vi "输入数据解析.vi"(0 "单个参数补充":dbl, 1 "从板号":dbl=1.0, 2 "主板二维码":string="BNET01", 3 "从板二维码":string="BNET01", 5 "主板引用":refnum<vi>, 7 "从板引用":refnum<vi>, 9 "主板选项":string="三级故障阀值", 11 "枚举":enum16{"主板", "从板"}(ring), 12 "快换":bool caption="快换写入") -> (4 "输出数组":dbl[][](array[numeric]), 6 "数组长度":dbl[](array[numeric]), 8 "循环次数":i32, 10 "命令":u32, 14 "名称":string[](array[string]), 15 "命令序号":u32[](array[numeric]))   [LabVIEW 2013] (continued)
                    n7568 = Quotient & Remainder(x=w19474, y=w19492) -> (x-y*floor(x/y)=w19491:dbl, floor(x/y)=w19495:dbl)
                    n7569 = Quotient & Remainder(x=w19473, y=w19487) -> (x-y*floor(x/y)=w19483:dbl, floor(x/y)=w19484:dbl)
                    n7570 = Quotient & Remainder(x=w19495, y=w19492) -> (x-y*floor(x/y)=w19490:dbl, floor(x/y)=w19494:dbl)
                    n7571 = Quotient & Remainder(x=w19484, y=w19487) -> (x-y*floor(x/y)=w19482:dbl, floor(x/y)=w19485:dbl)
                    n7572 = Quotient & Remainder(x=w19494, y=w19492) -> (x-y*floor(x/y)=w19489:dbl, floor(x/y)=w19493:dbl)
                    n7573 = Quotient & Remainder(x=w19485, y=w19487) -> (x-y*floor(x/y)=w19481:dbl, floor(x/y)=w19486:dbl)
                    n7574 = Quotient & Remainder(x=w19493, y=w19492) -> (x-y*floor(x/y)=w19488:dbl)  [unwired: 1 out]
                    n7575 = Quotient & Remainder(x=w19486, y=w19487) -> (x-y*floor(x/y)=w19480:dbl)  [unwired: 1 out]
                    n7576 = Build Array(w19488, w19489, w19490, w19491, w19480, w19481, w19482, w19483) -> (w19496:dbl[])
                  }
                  frame 3 {
                    w19504 = 256.0 ("y")
                    # "充电次数"
                    n7577 = Unbundle By Name(w19509) -> ("充电次数"=w19508:dbl, "应用车型"=w19506:dbl, "电池包组号"=w19505:dbl)
                    n7578 = Quotient & Remainder(x=w19508, y=w19504) -> (x-y*floor(x/y)=w19510:dbl, floor(x/y)=w19507:dbl)
                    n7579 = Quotient & Remainder(x=w19506, y=w19504) -> (x-y*floor(x/y)=w19502:dbl, floor(x/y)=w19503:dbl)
                    n7580 = Quotient & Remainder(x=w19505, y=w19504) -> (x-y*floor(x/y)=w19500:dbl, floor(x/y)=w19501:dbl)
                    n7581 = Build Array(w19507, w19510, w19503, w19502, w19501, w19500) -> (w19511:dbl[])
                  }
                  frame 4 {
                    # "SOC"
                    n7582 = Unbundle By Name(w19520) -> ("SOC"=w19519:dbl)
                    n7583 = call "输入分辨率计算-EV05.vi"("1字节?"=FALSE, "数值"=w19519, "分辨率"=0.1) -> ("低字节"=w19515:dbl, "高字节1"=w19516:dbl)  [unwired: 2 in, 5 out]
                    n7584 = Build Array(w19516, w19515) -> (w19521:dbl[])
                  }
                  frame 5 {
                    # "车牌号"
                    n7585 = Unbundle By Name(w19528) -> ("车牌号"=w19527:string)
                    n7586 = String To Byte Array(string=w19527) -> (unsigned byte array=w19531:u8[])
                    n7587 = Array Subset(array=w19531, length=8 ("长度")) -> (w19526:u8[])  [unwired: 1 in]
                  }
                  frame 6 {
                    n7588 = Unbundle By Name(w19549) -> ("最大允许单体电压"=w19547:dbl, "最大允许总电压"=w19546:dbl, "最大允许温度"=w19545:dbl, "最小允许温度"=w19544:dbl, "最大允许充电电流"=w19543:dbl, "最小允许充电电流"=w19542:dbl, "电流步长"=w19538:dbl, "最小允许单体电压"=w19541:dbl)
                    n7589 = call "输入分辨率计算-EV05.vi"("1字节?"=FALSE, "数值 2"=w19541, "数值"=w19547, "分辨率"=0.001) -> ("低字节 2"=w19533:dbl, "高字节 2"=w19534:dbl, "低字节"=w19557:dbl, "高字节1"=w19558:dbl)  [unwired: 1 in, 3 out]
                    n7590 = call "输入分辨率计算-EV05.vi"("1字节?"=FALSE, "数值"=w19546, "分辨率"=0.1) -> ("低字节"=w19555:dbl, "高字节1"=w19556:dbl)  [unwired: 2 in, 5 out]
                    n7591 = call "输入分辨率计算-EV05.vi"("1字节?"=TRUE, "数值 2"=w19544, "数值"=w19545, "偏移量"=-40.0, "分辨率"=1.0) -> ("高字节 2"=w19550:dbl, "高字节1"=w19554:dbl)  [unwired: 5 out]
                    n7592 = call "输入分辨率计算-EV05.vi"("1字节?"=FALSE, "数值 2"=w19542, "数值"=w19543, "偏移量"=0.0, "分辨率"=0.1) -> ("低字节 2"=w19539:dbl, "高字节 2"=w19540:dbl, "低字节"=w19552:dbl, "高字节1"=w19553:dbl)  [unwired: 3 out]
                    n7593 = Quotient & Remainder(x=w19538, y=256.0) -> (x-y*floor(x/y)=w19535:dbl, floor(x/y)=w19536:dbl)
                    n7594 = Build Array(w19558, w19557, w19556, w19555, w19554, w19550, w19553, w19552, w19540, w19539, w19536, w19535, w19534, w19533) -> (w19551:dbl[])
                  }
                }
              }
            }
          }
        }
        frame "电池包序号" {
          n7595 = case shown="真" w19573 {
            tunnel: [_ w19584] -> w19577
            tunnel: [_ w19583] -> w19576
            tunnel: w19575 -> [_ w19579]
            tunnel: [_ w19582] -> w19574
            tunnel: [_ u32 35 ("命令序号")] -> w19572
            frame False {
            }
            frame True {
              n7596 = Unbundle By Name(w19579) -> ("电池组信息(从板)"=w19580:refnum<vi>)
              n7597 = property class="Clust (严格)"(reference=w19580) -> ("Value"=w19578:T9)  [unwired: 1 in, 2 out]
              n7598 = for {
                N: 1 -> [_]
                tunnel: [w19590] -> w19584 mode=indexing
                tunnel: [w19589] -> w19583 mode=indexing
                tunnel: w19578 -> [w19588]
                tunnel: [w19587] -> w19582 mode=indexing
                i -> [w19586]
                n7599 = case shown="0, 默认" w19586 {
                  tunnel: [4 ("单个参数补充") 30 ("单个参数补充") 8 ("单个参数补充") 6 ("单个参数补充") 4 ("单个参数补充") 8 ("单个参数补充") 14 ("单个参数补充")] -> w19590
                  tunnel: [u32 2 ("命令序号") u32 1 ("命令序号") u32 3 ("命令序号") u32 4 ("命令序号") u32 5 ("命令序号") u32 6 ("命令序号") u32 7 ("命令序号")] -> w19589
                  tunnel: w19588 -> [w19598 w19614 w19626 w19655 w19665 w19672 w19692]
                  tunnel: [w19591 w19616 w19643 w19657 w19666 w19670 w19694] -> w19587
                  frame 0, Default {
                    n7600 = Unbundle By Name(w19598) -> ("电池包序号"=w19595:dbl)
                    n7601 = Quotient & Remainder(x=w19595, y=256.0) -> (x-y*floor(x/y)=w19592:dbl, floor(x/y)=w19593:dbl)
                    n7602 = Build Array(w19593, w19592) -> (w19591:dbl[])
                  }
                  frame 1 {
                    w19604 = 0 ("索引")
                    # "电池组信息"
                    n7603 = Unbundle By Name(w19614) -> ("电池类型"=w19606:dbl, "电池厂家"=w19605:dbl, "电池厂家"=w19607:dbl, "电池类型"=w19608:dbl, "额定能量"=w19612:dbl, "额定容量"=w19609:dbl, "实际容量"=w19601:dbl)
                    n7604 = Build Array(w19606, w19605, w19604, w19604, w19604, w19604, w19604, w19607, w19608) -> (w19603:dbl[])
                    n7605 = call "输入分辨率计算-EV05.vi"("1字节?"=FALSE, "数值"=w19601, "分辨率"=0.1) -> ("高字节1"=w19599:dbl)  [unwired: 2 in, 6 out]
                    n7606 = Quotient & Remainder(x=w19612, y=256.0) -> (x-y*floor(x/y)=w19610:dbl, floor(x/y)=w19611:dbl)
                    n7607 = call "电池组信息组合.vi"("数组"=w19603) -> ("电池信息组合"=w19617:dbl[])
                    n7608 = Insert Into Array(array=w19617, index=0 ("索引"), new element #1=w19611, new element #2=w19610, new element #3=w19609, new element #4=w19599, new element #5=w19599) -> (w19616:dbl[])
                  }
                  frame 2 {
                    w19634 = 256.0 ("y")
                    w19639 = 256.0 ("y")
                    # "充放电安时/安时数"
                    n7609 = Unbundle By Name(w19626) -> ("充电总安时"=w19623:dbl, "放电总这时"=w19622:dbl)
                    n7610 = call "输入分辨率计算-EV05.vi"("1字节?"=TRUE, "数值 2"=w19622, "数值"=w19623, "分辨率"=0.001) -> ("高字节 2"=w19620:dbl, "高字节1"=w19621:dbl)  [unwired: 1 in, 5 out]
                    n7611 = Quotient & Remainder(x=w19621, y=w19639) -> (x-y*floor(x/y)=w19638:dbl, floor(x/y)=w19642:dbl)
                    n7612 = Quotient & Remainder(x=w19620, y=w19634) -> (x-y*floor(x/y)=w19630:dbl, floor(x/y)=w19631:dbl)
                    n7613 = Quotient & Remainder(x=w19642, y=w19639) -> (x-y*floor(x/y)=w19637:dbl, floor(x/y)=w19641:dbl)
                    n7614 = Quotient & Remainder(x=w19631, y=w19634) -> (x-y*floor(x/y)=w19629:dbl, floor(x/y)=w19632:dbl)
                    n7615 = Quotient & Remainder(x=w19641, y=w19639) -> (x-y*floor(x/y)=w19636:dbl, floor(x/y)=w19640:dbl)
                    n7616 = Quotient & Remainder(x=w19632, y=w19634) -> (x-y*floor(x/y)=w19628:dbl, floor(x/y)=w19633:dbl)
                    n7617 = Quotient & Remainder(x=w19640, y=w19639) -> (x-y*floor(x/y)=w19635:dbl)  [unwired: 1 out]
                    n7618 = Quotient & Remainder(x=w19633, y=w19634) -> (x-y*floor(x/y)=w19627:dbl)  [unwired: 1 out]
                    n7619 = Build Array(w19635, w19636, w19637, w19638, w19627, w19628, w19629, w19630) -> (w19643:dbl[])
                  }
                  frame 3 {
                    w19650 = 256.0 ("y")
                    # "充电次数"
                    n7620 = Unbundle By Name(w19655) -> ("充电次数"=w19654:dbl, "应用车型"=w19652:dbl, "电池包组号"=w19651:dbl)
                    n7621 = Quotient & Remainder(x=w19654, y=w19650) -> (x-y*floor(x/y)=w19656:dbl, floor(x/y)=w19653:dbl)
                    n7622 = Quotient & Remainder(x=w19652, y=w19650) -> (x-y*floor(x/y)=w19648:dbl, floor(x/y)=w19649:dbl)
                    n7623 = Quotient & Remainder(x=w19651, y=w19650) -> (x-y*floor(x/y)=w19646:dbl, floor(x/y)=w19647:dbl)
                    n7624 = Build Array(w19653, w19656, w19649, w19648, w19647, w19646) -> (w19657:dbl[])
                  }
                  frame 4 {
                    # "SOC"
                    n7625 = Unbundle By Name(w19665) -> ("SOC"=w19664:dbl)
                    n7626 = call "输入分辨率计算-EV05.vi"("1字节?"=FALSE, "数值"=w19664, "分辨率"=0.1) -> ("低字节"=w19660:dbl, "高字节1"=w19661:dbl)  [unwired: 2 in, 5 out]
                    n7627 = Build Array(w19661, w19660) -> (w19666:dbl[])
                  }
                  frame 5 {
                    # "车牌号"
                    n7628 = Unbundle By Name(w19672) -> ("车牌号"=w19671:string)
                    n7629 = String To Byte Array(string=w19671) -> (unsigned byte array=w19675:u8[])
                    n7630 = Array Subset(array=w19675, length=8 ("长度")) -> (w19670:u8[])  [unwired: 1 in]
                  }
                  frame 6 {
                    n7631 = Unbundle By Name(w19692) -> ("最大允许单体电压"=w19690:dbl, "最大允许总电压"=w19689:dbl, "最大允许温度"=w19688:dbl, "最小允许温度"=w19687:dbl, "最大允许充电电流"=w19686:dbl, "最小允许充电电流"=w19685:dbl, "电流步长"=w19681:dbl, "最小允许单体电压"=w19684:dbl)
                    n7632 = call "输入分辨率计算-EV05.vi"("1字节?"=FALSE, "数值 2"=w19684, "数值"=w19690, "分辨率"=0.001) -> ("低字节 2"=w19676:dbl, "高字节 2"=w19677:dbl, "低字节"=w19700:dbl, "高字节1"=w19701:dbl)  [unwired: 1 in, 3 out]
                    n7633 = call "输入分辨率计算-EV05.vi"("1字节?"=FALSE, "数值"=w19689, "分辨率"=0.1) -> ("低字节"=w19698:dbl, "高字节1"=w19699:dbl)  [unwired: 2 in, 5 out]
                    n7634 = call "输入分辨率计算-EV05.vi"("1字节?"=TRUE, "数值 2"=w19687, "数值"=w19688, "偏移量"=-40.0, "分辨率"=1.0) -> ("高字节 2"=w19693:dbl, "高字节1"=w19697:dbl)  [unwired: 5 out]
                    n7635 = call "输入分辨率计算-EV05.vi"("1字节?"=FALSE, "数值 2"=w19685, "数值"=w19686, "偏移量"=0.0, "分辨率"=0.1) -> ("低字节 2"=w19682:dbl, "高字节 2"=w19683:dbl, "低字节"=w19695:dbl, "高字节1"=w19696:dbl)  [unwired: 3 out]
                    n7636 = Quotient & Remainder(x=w19681, y=256.0) -> (x-y*floor(x/y)=w19678:dbl, floor(x/y)=w19679:dbl)
                    n7637 = Build Array(w19701, w19700, w19699, w19698, w19697, w19693, w19696, w19695, w19683, w19682, w19679, w19678, w19677, w19676) -> (w19694:dbl[])
                  }
                }
              }
            }
          }
        }
        frame "充放电安时" {
          n7638 = case shown="真" w19716 {
            tunnel: [_ w19727] -> w19720
            tunnel: [_ w19726] -> w19719
            tunnel: w19718 -> [_ w19722]
            tunnel: [_ w19725] -> w19717
            tunnel: [_ u32 35 ("命令序号")] -> w19715
            frame False {
            }
            frame True {
              n7639 = Unbundle By Name(w19722) -> ("电池组信息(从板)"=w19723:refnum<vi>)
              n7640 = property class="Clust (严格)"(reference=w19723) -> ("Value"=w19721:T9)  [unwired: 1 in, 2 out]
              n7641 = for {
                N: 1 -> [_]
                tunnel: [w19733] -> w19727 mode=indexing
                tunnel: [w19732] -> w19726 mode=indexing
                tunnel: w19721 -> [w19731]
                tunnel: [w19730] -> w19725 mode=indexing
                i -> [w19729]
                n7642 = case shown="0, 默认" w19729 {
                  tunnel: [8 ("单个参数补充") 30 ("单个参数补充") 4 ("单个参数补充") 6 ("单个参数补充") 4 ("单个参数补充") 8 ("单个参数补充") 14 ("单个参数补充")] -> w19733
                  tunnel: [u32 3 ("命令序号") u32 1 ("命令序号") u32 2 ("命令序号") u32 4 ("命令序号") u32 5 ("命令序号") u32 6 ("命令序号") u32 7 ("命令序号")] -> w19732
                  tunnel: w19731 -> [w19740 w19775 w19788 w19798 w19808 w19815 w19835]
                  tunnel: [w19757 w19777 w19781 w19800 w19809 w19813 w19837] -> w19730
                  frame 0, Default {
                    w19748 = 256.0 ("y")
                    w19753 = 256.0 ("y")
                    # "充放电安时/安时数"
                    n7643 = Unbundle By Name(w19740) -> ("充电总安时"=w19737:dbl, "放电总这时"=w19736:dbl)
                    n7644 = call "输入分辨率计算-EV05.vi"("1字节?"=TRUE, "数值 2"=w19736, "数值"=w19737, "分辨率"=0.001) -> ("高字节 2"=w19734:dbl, "高字节1"=w19735:dbl)  [unwired: 1 in, 5 out]
                    n7645 = Quotient & Remainder(x=w19735, y=w19753) -> (x-y*floor(x/y)=w19752:dbl, floor(x/y)=w19756:dbl)
                    n7646 = Quotient & Remainder(x=w19734, y=w19748) -> (x-y*floor(x/y)=w19744:dbl, floor(x/y)=w19745:dbl)
                    n7647 = Quotient & Remainder(x=w19756, y=w19753) -> (x-y*floor(x/y)=w19751:dbl, floor(x/y)=w19755:dbl)
                    n7648 = Quotient & Remainder(x=w19745, y=w19748) -> (x-y*floor(x/y)=w19743:dbl, floor(x/y)=w19746:dbl)
                    n7649 = Quotient & Remainder(x=w19755, y=w19753) -> (x-y*floor(x/y)=w19750:dbl, floor(x/y)=w19754:dbl)
                    n7650 = Quotient & Remainder(x=w19746, y=w19748) -> (x-y*floor(x/y)=w19742:dbl, floor(x/y)=w19747:dbl)
                    n7651 = Quotient & Remainder(x=w19754, y=w19753) -> (x-y*floor(x/y)=w19749:dbl)  [unwired: 1 out]
                    n7652 = Quotient & Remainder(x=w19747, y=w19748) -> (x-y*floor(x/y)=w19741:dbl)  [unwired: 1 out]
                    n7653 = Build Array(w19749, w19750, w19751, w19752, w19741, w19742, w19743, w19744) -> (w19757:dbl[])
                  }
                  frame 1 {
                    w19765 = 0 ("索引")
                    # "电池组信息"
                    n7654 = Unbundle By Name(w19775) -> ("电池类型"=w19767:dbl, "电池厂家"=w19766:dbl, "电池厂家"=w19768:dbl, "电池类型"=w19769:dbl, "额定能量"=w19773:dbl, "额定容量"=w19770:dbl, "实际容量"=w19762:dbl)
                    n7655 = Build Array(w19767, w19766, w19765, w19765, w19765, w19765, w19765, w19768, w19769) -> (w19764:dbl[])
                    n7656 = call "输入分辨率计算-EV05.vi"("1字节?"=FALSE, "数值"=w19762, "分辨率"=0.1) -> ("高字节1"=w19760:dbl)  [unwired: 2 in, 6 out]
                    n7657 = Quotient & Remainder(x=w19773, y=256.0) -> (x-y*floor(x/y)=w19771:dbl, floor(x/y)=w19772:dbl)
                    n7658 = call "电池组信息组合.vi"("数组"=w19764) -> ("电池信息组合"=w19778:dbl[])
                    n7659 = Insert Into Array(array=w19778, index=0 ("索引"), new element #1=w19772, new element #2=w19771, new element #3=w19770, new element #4=w19760, new element #5=w19760) -> (w19777:dbl[])
                  }
                  frame 2 {
                    n7660 = Unbundle By Name(w19788) -> ("电池包序号"=w19785:dbl)
                    n7661 = Quotient & Remainder(x=w19785, y=256.0) -> (x-y*floor(x/y)=w19782:dbl, floor(x/y)=w19783:dbl)
                    n7662 = Build Array(w19783, w19782) -> (w19781:dbl[])
                  }
                  frame 3 {
                    w19793 = 256.0 ("y")
                    # "充电次数"
                    n7663 = Unbundle By Name(w19798) -> ("充电次数"=w19797:dbl, "应用车型"=w19795:dbl, "电池包组号"=w19794:dbl)
                    n7664 = Quotient & Remainder(x=w19797, y=w19793) -> (x-y*floor(x/y)=w19799:dbl, floor(x/y)=w19796:dbl)
                    n7665 = Quotient & Remainder(x=w19795, y=w19793) -> (x-y*floor(x/y)=w19791:dbl, floor(x/y)=w19792:dbl)
                    n7666 = Quotient & Remainder(x=w19794, y=w19793) -> (x-y*floor(x/y)=w19789:dbl, floor(x/y)=w19790:dbl)
                    n7667 = Build Array(w19796, w19799, w19792, w19791, w19790, w19789) -> (w19800:dbl[])
                  }
                  frame 4 {
                    # "SOC"
                    n7668 = Unbundle By Name(w19808) -> ("SOC"=w19807:dbl)
                    n7669 = call "输入分辨率计算-EV05.vi"("1字节?"=FALSE, "数值"=w19807, "分辨率"=0.1) -> ("低字节"=w19803:dbl, "高字节1"=w19804:dbl)  [unwired: 2 in, 5 out]
                    n7670 = Build Array(w19804, w19803) -> (w19809:dbl[])
                  }
                  frame 5 {
                    # "车牌号"
                    n7671 = Unbundle By Name(w19815) -> ("车牌号"=w19814:string)
                    n7672 = String To Byte Array(string=w19814) -> (unsigned byte array=w19818:u8[])
                    n7673 = Array Subset(array=w19818, length=8 ("长度")) -> (w19813:u8[])  [unwired: 1 in]
                  }
                  frame 6 {
                    n7674 = Unbundle By Name(w19835) -> ("最大允许单体电压"=w19833:dbl, "最大允许总电压"=w19832:dbl, "最大允许温度"=w19831:dbl, "最小允许温度"=w19830:dbl, "最大允许充电电流"=w19829:dbl, "最小允许充电电流"=w19828:dbl, "电流步长"=w19824:dbl, "最小允许单体电压"=w19827:dbl)
                    n7675 = call "输入分辨率计算-EV05.vi"("1字节?"=FALSE, "数值 2"=w19827, "数值"=w19833, "分辨率"=0.001) -> ("低字节 2"=w19819:dbl, "高字节 2"=w19820:dbl, "低字节"=w19843:dbl, "高字节1"=w19844:dbl)  [unwired: 1 in, 3 out]
                    n7676 = call "输入分辨率计算-EV05.vi"("1字节?"=FALSE, "数值"=w19832, "分辨率"=0.1) -> ("低字节"=w19841:dbl, "高字节1"=w19842:dbl)  [unwired: 2 in, 5 out]
                    n7677 = call "输入分辨率计算-EV05.vi"("1字节?"=TRUE, "数值 2"=w19830, "数值"=w19831, "偏移量"=-40.0, "分辨率"=1.0) -> ("高字节 2"=w19836:dbl, "高字节1"=w19840:dbl)  [unwired: 5 out]
                    n7678 = call "输入分辨率计算-EV05.vi"("1字节?"=FALSE, "数值 2"=w19828, "数值"=w19829, "偏移量"=0.0, "分辨率"=0.1) -> ("低字节 2"=w19825:dbl, "高字节 2"=w19826:dbl, "低字节"=w19838:dbl, "高字节1"=w19839:dbl)  [unwired: 3 out]
                    n7679 = Quotient & Remainder(x=w19824, y=256.0) -> (x-y*floor(x/y)=w19821:dbl, floor(x/y)=w19822:dbl)
                    n7680 = Build Array(w19844, w19843, w19842, w19841, w19840, w19836, w19839, w19838, w19826, w19825, w19822, w19821, w19820, w19819) -> (w19837:dbl[])
                  }
                }
              }
            }
          }
        }
        frame "充电次数时间" {
          n7681 = case shown="真" w19859 {
            tunnel: [_ w19870] -> w19863
            tunnel: [_ w19869] -> w19862
            tunnel: w19861 -> [_ w19865]
            tunnel: [_ w19868] -> w19860
            tunnel: [_ u32 35 ("命令序号")] -> w19858
            frame False {
            }
            frame True {
              n7682 = Unbundle By Name(w19865) -> ("电池组信息(从板)"=w19866:refnum<vi>)
              n7683 = property class="Clust (严格)"(reference=w19866) -> ("Value"=w19864:T9)  [unwired: 1 in, 2 out]
              n7684 = for {
                N: 1 -> [_]
                tunnel: [w19876] -> w19870 mode=indexing
                tunnel: [w19875] -> w19869 mode=indexing
                tunnel: w19864 -> [w19874]
                tunnel: [w19873] -> w19868 mode=indexing
                i -> [w19872]
                n7685 = case shown="0, 默认" w19872 {
                  tunnel: [6 ("单个参数补充") 30 ("单个参数补充") 4 ("单个参数补充") 8 ("单个参数补充") 4 ("单个参数补充") 8 ("单个参数补充") 14 ("单个参数补充")] -> w19876
                  tunnel: [u32 4 ("命令序号") u32 1 ("命令序号") u32 2 ("命令序号") u32 3 ("命令序号") u32 5 ("命令序号") u32 6 ("命令序号") u32 7 ("命令序号")] -> w19875
                  tunnel: w19874 -> [w19886 w19906 w19919 w19926 w19951 w19958 w19978]
                  tunnel: [w19888 w19908 w19912 w19943 w19952 w19956 w19980] -> w19873
                  frame 0, Default {
                    w19881 = 256.0 ("y")
                    # "充电次数"
                    n7686 = Unbundle By Name(w19886) -> ("放空次数"=w19885:dbl, "充满次数"=w19883:dbl, "充电次数"=w19882:dbl)
                    n7687 = Quotient & Remainder(x=w19885, y=w19881) -> (x-y*floor(x/y)=w19887:dbl, floor(x/y)=w19884:dbl)
                    n7688 = Quotient & Remainder(x=w19883, y=w19881) -> (x-y*floor(x/y)=w19879:dbl, floor(x/y)=w19880:dbl)
                    n7689 = Quotient & Remainder(x=w19882, y=w19881) -> (x-y*floor(x/y)=w19877:dbl, floor(x/y)=w19878:dbl)
                    n7690 = Build Array(w19884, w19887, w19880, w19879, w19878, w19877) -> (w19888:dbl[])
                  }
                  frame 1 {
                    w19896 = 0 ("索引")
                    # "电池组信息"
                    n7691 = Unbundle By Name(w19906) -> ("电池类型"=w19898:dbl, "电池厂家"=w19897:dbl, "电池厂家"=w19899:dbl, "电池类型"=w19900:dbl, "额定能量"=w19904:dbl, "额定容量"=w19901:dbl, "实际容量"=w19893:dbl)
                    n7692 = Build Array(w19898, w19897, w19896, w19896, w19896, w19896, w19896, w19899, w19900) -> (w19895:dbl[])
                    n7693 = call "输入分辨率计算-EV05.vi"("1字节?"=FALSE, "数值"=w19893, "分辨率"=0.1) -> ("高字节1"=w19891:dbl)  [unwired: 2 in, 6 out]
                    n7694 = Quotient & Remainder(x=w19904, y=256.0) -> (x-y*floor(x/y)=w19902:dbl, floor(x/y)=w19903:dbl)
                    n7695 = call "电池组信息组合.vi"("数组"=w19895) -> ("电池信息组合"=w19909:dbl[])
                    n7696 = Insert Into Array(array=w19909, index=0 ("索引"), new element #1=w19903, new element #2=w19902, new element #3=w19901, new element #4=w19891, new element #5=w19891) -> (w19908:dbl[])
                  }
                  frame 2 {
                    n7697 = Unbundle By Name(w19919) -> ("电池包序号"=w19916:dbl)
                    n7698 = Quotient & Remainder(x=w19916, y=256.0) -> (x-y*floor(x/y)=w19913:dbl, floor(x/y)=w19914:dbl)
                    n7699 = Build Array(w19914, w19913) -> (w19912:dbl[])
                  }
                  frame 3 {
                    w19934 = 256.0 ("y")
                    w19939 = 256.0 ("y")
                    # "充放电安时/安时数"
                    n7700 = Unbundle By Name(w19926) -> ("充电总安时"=w19923:dbl, "放电总这时"=w19922:dbl)
                    n7701 = call "输入分辨率计算-EV05.vi"("1字节?"=TRUE, "数值 2"=w19922, "数值"=w19923, "分辨率"=0.001) -> ("高字节 2"=w19920:dbl, "高字节1"=w19921:dbl)  [unwired: 1 in, 5 out]
                    n7702 = Quotient & Remainder(x=w19921, y=w19939) -> (x-y*floor(x/y)=w19938:dbl, floor(x/y)=w19942:dbl)
                    n7703 = Quotient & Remainder(x=w19920, y=w19934) -> (x-y*floor(x/y)=w19930:dbl, floor(x/y)=w19931:dbl)
                    n7704 = Quotient & Remainder(x=w19942, y=w19939) -> (x-y*floor(x/y)=w19937:dbl, floor(x/y)=w19941:dbl)
                    n7705 = Quotient & Remainder(x=w19931, y=w19934) -> (x-y*floor(x/y)=w19929:dbl, floor(x/y)=w19932:dbl)
                    n7706 = Quotient & Remainder(x=w19941, y=w19939) -> (x-y*floor(x/y)=w19936:dbl, floor(x/y)=w19940:dbl)
                    n7707 = Quotient & Remainder(x=w19932, y=w19934) -> (x-y*floor(x/y)=w19928:dbl, floor(x/y)=w19933:dbl)
                    n7708 = Quotient & Remainder(x=w19940, y=w19939) -> (x-y*floor(x/y)=w19935:dbl)  [unwired: 1 out]
                    n7709 = Quotient & Remainder(x=w19933, y=w19934) -> (x-y*floor(x/y)=w19927:dbl)  [unwired: 1 out]
                    n7710 = Build Array(w19935, w19936, w19937, w19938, w19927, w19928, w19929, w19930) -> (w19943:dbl[])
                  }
                  frame 4 {
                    # "SOC"
                    n7711 = Unbundle By Name(w19951) -> ("SOC"=w19950:dbl)
                    n7712 = call "输入分辨率计算-EV05.vi"("1字节?"=FALSE, "数值"=w19950, "分辨率"=0.1) -> ("低字节"=w19946:dbl, "高字节1"=w19947:dbl)  [unwired: 2 in, 5 out]
                    n7713 = Build Array(w19947, w19946) -> (w19952:dbl[])
                  }
                  frame 5 {
                    # "车牌号"
                    n7714 = Unbundle By Name(w19958) -> ("车牌号"=w19957:string)
                    n7715 = String To Byte Array(string=w19957) -> (unsigned byte array=w19961:u8[])
                    n7716 = Array Subset(array=w19961, length=8 ("长度")) -> (w19956:u8[])  [unwired: 1 in]
                  }
                  frame 6 {
                    n7717 = Unbundle By Name(w19978) -> ("最大允许单体电压"=w19976:dbl, "最大允许总电压"=w19975:dbl, "最大允许温度"=w19974:dbl, "最小允许温度"=w19973:dbl, "最大允许充电电流"=w19972:dbl, "最小允许充电电流"=w19971:dbl, "电流步长"=w19967:dbl, "最小允许单体电压"=w19970:dbl)
                    n7718 = call "输入分辨率计算-EV05.vi"("1字节?"=FALSE, "数值 2"=w19970, "数值"=w19976, "分辨率"=0.001) -> ("低字节 2"=w19962:dbl, "高字节 2"=w19963:dbl, "低字节"=w19986:dbl, "高字节1"=w19987:dbl)  [unwired: 1 in, 3 out]
                    n7719 = call "输入分辨率计算-EV05.vi"("1字节?"=FALSE, "数值"=w19975, "分辨率"=0.1) -> ("低字节"=w19984:dbl, "高字节1"=w19985:dbl)  [unwired: 2 in, 5 out]
                    n7720 = call "输入分辨率计算-EV05.vi"("1字节?"=TRUE, "数值 2"=w19973, "数值"=w19974, "偏移量"=-40.0, "分辨率"=1.0) -> ("高字节 2"=w19979:dbl, "高字节1"=w19983:dbl)  [unwired: 5 out]
                    n7721 = call "输入分辨率计算-EV05.vi"("1字节?"=FALSE, "数值 2"=w19971, "数值"=w19972, "偏移量"=0.0, "分辨率"=0.1) -> ("低字节 2"=w19968:dbl, "高字节 2"=w19969:dbl, "低字节"=w19981:dbl, "高字节1"=w19982:dbl)  [unwired: 3 out]
                    n7722 = Quotient & Remainder(x=w19967, y=256.0) -> (x-y*floor(x/y)=w19964:dbl, floor(x/y)=w19965:dbl)
                    n7723 = Build Array(w19987, w19986, w19985, w19984, w19983, w19979, w19982, w19981, w19969, w19968, w19965, w19964, w19963, w19962) -> (w19980:dbl[])
                  }
                }
              }
            }
          }
        }
        frame "SOC" {
          n7724 = case shown="真" w20002 {
            tunnel: [_ w20013] -> w20006
            tunnel: [_ w20012] -> w20005
            tunnel: w20004 -> [_ w20008]
            tunnel: [_ w20011] -> w20003
            tunnel: [_ u32 35 ("命令序号")] -> w20001
            frame False {
            }
            frame True {
              n7725 = Unbundle By Name(w20008) -> ("电池组信息(从板)"=w20009:refnum<vi>)
              n7726 = property class="Clust (严格)"(reference=w20009) -> ("Value"=w20007:T9)  [unwired: 1 in, 2 out]
              n7727 = for {
                N: 1 -> [_]
                tunnel: [w20019] -> w20013 mode=indexing
                tunnel: [w20018] -> w20012 mode=indexing
                tunnel: w20007 -> [w20017]
                tunnel: [w20016] -> w20011 mode=indexing
                i -> [w20015]
                n7728 = case shown="0, 默认" w20015 {
                  tunnel: [2 ("单个参数补充") 30 ("单个参数补充") 4 ("单个参数补充") 8 ("单个参数补充") 6 ("单个参数补充") 8 ("单个参数补充") 14 ("单个参数补充")] -> w20019
                  tunnel: [u32 5 ("命令序号") u32 1 ("命令序号") u32 2 ("命令序号") u32 3 ("命令序号") u32 4 ("命令序号") u32 6 ("命令序号") u32 7 ("命令序号")] -> w20018
                  tunnel: w20017 -> [w20025 w20044 w20057 w20064 w20093 w20101 w20121]
                  tunnel: [w20026 w20046 w20050 w20081 w20095 w20099 w20123] -> w20016
                  frame 0, Default {
                    # "SOC"
                    n7729 = Unbundle By Name(w20025) -> ("SOC"=w20024:dbl)
                    n7730 = call "输入分辨率计算-EV05.vi"("1字节?"=FALSE, "数值"=w20024, "分辨率"=0.1) -> ("低字节"=w20020:dbl, "高字节1"=w20021:dbl)  [unwired: 2 in, 5 out]
                    n7731 = Build Array(w20021, w20020) -> (w20026:dbl[])
                  }
                  frame 1 {
                    w20034 = 0 ("索引")
                    # "电池组信息"
                    n7732 = Unbundle By Name(w20044) -> ("电池类型"=w20036:dbl, "电池厂家"=w20035:dbl, "电池厂家"=w20037:dbl, "电池类型"=w20038:dbl, "额定能量"=w20042:dbl, "额定容量"=w20039:dbl, "实际容量"=w20031:dbl)
                    n7733 = Build Array(w20036, w20035, w20034, w20034, w20034, w20034, w20034, w20037, w20038) -> (w20033:dbl[])
                    n7734 = call "输入分辨率计算-EV05.vi"("1字节?"=FALSE, "数值"=w20031, "分辨率"=0.1) -> ("高字节1"=w20029:dbl)  [unwired: 2 in, 6 out]
                    n7735 = Quotient & Remainder(x=w20042, y=256.0) -> (x-y*floor(x/y)=w20040:dbl, floor(x/y)=w20041:dbl)
                    n7736 = call "电池组信息组合.vi"("数组"=w20033) -> ("电池信息组合"=w20047:dbl[])
                    n7737 = Insert Into Array(array=w20047, index=0 ("索引"), new element #1=w20041, new element #2=w20040, new element #3=w20039, new element #4=w20029, new element #5=w20029) -> (w20046:dbl[])
                  }
                  frame 2 {
                    n7738 = Unbundle By Name(w20057) -> ("电池包序号"=w20054:dbl)
                    n7739 = Quotient & Remainder(x=w20054, y=256.0) -> (x-y*floor(x/y)=w20051:dbl, floor(x/y)=w20052:dbl)
                    n7740 = Build Array(w20052, w20051) -> (w20050:dbl[])
                  }
                  frame 3 {
                    w20072 = 256.0 ("y")
                    w20077 = 256.0 ("y")
                    # "充放电安时/安时数"
                    n7741 = Unbundle By Name(w20064) -> ("充电总安时"=w20061:dbl, "放电总这时"=w20060:dbl)
                    n7742 = call "输入分辨率计算-EV05.vi"("1字节?"=TRUE, "数值 2"=w20060, "数值"=w20061, "分辨率"=0.001) -> ("高字节 2"=w20058:dbl, "高字节1"=w20059:dbl)  [unwired: 1 in, 5 out]
                    n7743 = Quotient & Remainder(x=w20059, y=w20077) -> (x-y*floor(x/y)=w20076:dbl, floor(x/y)=w20080:dbl)
                    n7744 = Quotient & Remainder(x=w20058, y=w20072) -> (x-y*floor(x/y)=w20068:dbl, floor(x/y)=w20069:dbl)
                    n7745 = Quotient & Remainder(x=w20080, y=w20077) -> (x-y*floor(x/y)=w20075:dbl, floor(x/y)=w20079:dbl)
                    n7746 = Quotient & Remainder(x=w20069, y=w20072) -> (x-y*floor(x/y)=w20067:dbl, floor(x/y)=w20070:dbl)
                    n7747 = Quotient & Remainder(x=w20079, y=w20077) -> (x-y*floor(x/y)=w20074:dbl, floor(x/y)=w20078:dbl)
                    n7748 = Quotient & Remainder(x=w20070, y=w20072) -> (x-y*floor(x/y)=w20066:dbl, floor(x/y)=w20071:dbl)
                    n7749 = Quotient & Remainder(x=w20078, y=w20077) -> (x-y*floor(x/y)=w20073:dbl)  [unwired: 1 out]
                    n7750 = Quotient & Remainder(x=w20071, y=w20072) -> (x-y*floor(x/y)=w20065:dbl)  [unwired: 1 out]
                    n7751 = Build Array(w20073, w20074, w20075, w20076, w20065, w20066, w20067, w20068) -> (w20081:dbl[])
                  }
                  frame 4 {
                    w20088 = 256.0 ("y")
                    # "充电次数"
                    n7752 = Unbundle By Name(w20093) -> ("充电次数"=w20092:dbl, "应用车型"=w20090:dbl, "电池包组号"=w20089:dbl)
                    n7753 = Quotient & Remainder(x=w20092, y=w20088) -> (x-y*floor(x/y)=w20094:dbl, floor(x/y)=w20091:dbl)
                    n7754 = Quotient & Remainder(x=w20090, y=w20088) -> (x-y*floor(x/y)=w20086:dbl, floor(x/y)=w20087:dbl)
                    n7755 = Quotient & Remainder(x=w20089, y=w20088) -> (x-y*floor(x/y)=w20084:dbl, floor(x/y)=w20085:dbl)
                    n7756 = Build Array(w20091, w20094, w20087, w20086, w20085, w20084) -> (w20095:dbl[])
                  }
                  frame 5 {
                    # "车牌号"
                    n7757 = Unbundle By Name(w20101) -> ("车牌号"=w20100:string)
                    n7758 = String To Byte Array(string=w20100) -> (unsigned byte array=w20104:u8[])
                    n7759 = Array Subset(array=w20104, length=8 ("长度")) -> (w20099:u8[])  [unwired: 1 in]
                  }
                  frame 6 {
                    n7760 = Unbundle By Name(w20121) -> ("最大允许单体电压"=w20119:dbl, "最大允许总电压"=w20118:dbl, "最大允许温度"=w20117:dbl, "最小允许温度"=w20116:dbl, "最大允许充电电流"=w20115:dbl, "最小允许充电电流"=w20114:dbl, "电流步长"=w20110:dbl, "最小允许单体电压"=w20113:dbl)
                    n7761 = call "输入分辨率计算-EV05.vi"("1字节?"=FALSE, "数值 2"=w20113, "数值"=w20119, "分辨率"=0.001) -> ("低字节 2"=w20105:dbl, "高字节 2"=w20106:dbl, "低字节"=w20129:dbl, "高字节1"=w20130:dbl)  [unwired: 1 in, 3 out]
                    n7762 = call "输入分辨率计算-EV05.vi"("1字节?"=FALSE, "数值"=w20118, "分辨率"=0.1) -> ("低字节"=w20127:dbl, "高字节1"=w20128:dbl)  [unwired: 2 in, 5 out]
                    n7763 = call "输入分辨率计算-EV05.vi"("1字节?"=TRUE, "数值 2"=w20116, "数值"=w20117, "偏移量"=-40.0, "分辨率"=1.0) -> ("高字节 2"=w20122:dbl, "高字节1"=w20126:dbl)  [unwired: 5 out]
                    n7764 = call "输入分辨率计算-EV05.vi"("1字节?"=FALSE, "数值 2"=w20114, "数值"=w20115, "偏移量"=0.0, "分辨率"=0.1) -> ("低字节 2"=w20111:dbl, "高字节 2"=w20112:dbl, "低字节"=w20124:dbl, "高字节1"=w20125:dbl)  [unwired: 3 out]
                    n7765 = Quotient & Remainder(x=w20110, y=256.0) -> (x-y*floor(x/y)=w20107:dbl, floor(x/y)=w20108:dbl)
                    n7766 = Build Array(w20130, w20129, w20128, w20127, w20126, w20122, w20125, w20124, w20112, w20111, w20108, w20107, w20106, w20105) -> (w20123:dbl[])
                  }
                }
              }
            }
          }
        }
        frame "车牌号" {
          n7767 = case shown="真" w20145 {
            tunnel: [_ w20156] -> w20149
            tunnel: [_ w20155] -> w20148
            tunnel: w20147 -> [_ w20151]
            tunnel: [_ w20154] -> w20146
            tunnel: [_ u32 35 ("命令序号")] -> w20144
            frame False {
            }
            frame True {
              n7768 = Unbundle By Name(w20151) -> ("电池组信息(从板)"=w20152:refnum<vi>)
              n7769 = property class="Clust (严格)"(reference=w20152) -> ("Value"=w20150:T9)  [unwired: 1 in, 2 out]
              n7770 = for {
                N: 1 -> [_]
                tunnel: [w20162] -> w20156 mode=indexing
                tunnel: [w20161] -> w20155 mode=indexing
                tunnel: w20150 -> [w20160]
                tunnel: [w20159] -> w20154 mode=indexing
                i -> [w20158]
                n7771 = case shown="0, 默认" w20158 {
                  tunnel: [8 ("单个参数补充") 30 ("单个参数补充") 4 ("单个参数补充") 8 ("单个参数补充") 6 ("单个参数补充") 4 ("单个参数补充") 14 ("单个参数补充")] -> w20162
                  tunnel: [u32 6 ("命令序号") u32 1 ("命令序号") u32 2 ("命令序号") u32 3 ("命令序号") u32 4 ("命令序号") u32 5 ("命令序号") u32 7 ("命令序号")] -> w20161
                  tunnel: w20160 -> [w20166 w20185 w20198 w20205 w20234 w20244 w20264]
                  tunnel: [w20164 w20187 w20191 w20222 w20236 w20245 w20266] -> w20159
                  frame 0, Default {
                    # "车牌号"
                    n7772 = Unbundle By Name(w20166) -> ("车牌号"=w20165:string)
                    n7773 = String To Byte Array(string=w20165) -> (unsigned byte array=w20169:u8[])
                    n7774 = Array Subset(array=w20169, length=8 ("长度")) -> (w20164:u8[])  [unwired: 1 in]
                  }
                  frame 1 {
                    w20175 = 0 ("索引")
                    # "电池组信息"
                    n7775 = Unbundle By Name(w20185) -> ("电池类型"=w20177:dbl, "电池厂家"=w20176:dbl, "电池厂家"=w20178:dbl, "电池类型"=w20179:dbl, "额定能量"=w20183:dbl, "额定容量"=w20180:dbl, "实际容量"=w20172:dbl)
                    n7776 = Build Array(w20177, w20176, w20175, w20175, w20175, w20175, w20175, w20178, w20179) -> (w20174:dbl[])
                    n7777 = call "输入分辨率计算-EV05.vi"("1字节?"=FALSE, "数值"=w20172, "分辨率"=0.1) -> ("高字节1"=w20170:dbl)  [unwired: 2 in, 6 out]
                    n7778 = Quotient & Remainder(x=w20183, y=256.0) -> (x-y*floor(x/y)=w20181:dbl, floor(x/y)=w20182:dbl)
                    n7779 = call "电池组信息组合.vi"("数组"=w20174) -> ("电池信息组合"=w20188:dbl[])
                    n7780 = Insert Into Array(array=w20188, index=0 ("索引"), new element #1=w20182, new element #2=w20181, new element #3=w20180, new element #4=w20170, new element #5=w20170) -> (w20187:dbl[])
                  }
                  frame 2 {
                    n7781 = Unbundle By Name(w20198) -> ("电池包序号"=w20195:dbl)
                    n7782 = Quotient & Remainder(x=w20195, y=256.0) -> (x-y*floor(x/y)=w20192:dbl, floor(x/y)=w20193:dbl)
                    n7783 = Build Array(w20193, w20192) -> (w20191:dbl[])
                  }
                  frame 3 {
                    w20213 = 256.0 ("y")
                    w20218 = 256.0 ("y")
                    # "充放电安时/安时数"
                    n7784 = Unbundle By Name(w20205) -> ("充电总安时"=w20202:dbl, "放电总这时"=w20201:dbl)
                    n7785 = call "输入分辨率计算-EV05.vi"("1字节?"=TRUE, "数值 2"=w20201, "数值"=w20202, "分辨率"=0.001) -> ("高字节 2"=w20199:dbl, "高字节1"=w20200:dbl)  [unwired: 1 in, 5 out]
                    n7786 = Quotient & Remainder(x=w20200, y=w20218) -> (x-y*floor(x/y)=w20217:dbl, floor(x/y)=w20221:dbl)
                    n7787 = Quotient & Remainder(x=w20199, y=w20213) -> (x-y*floor(x/y)=w20209:dbl, floor(x/y)=w20210:dbl)
                    n7788 = Quotient & Remainder(x=w20221, y=w20218) -> (x-y*floor(x/y)=w20216:dbl, floor(x/y)=w20220:dbl)
                    n7789 = Quotient & Remainder(x=w20210, y=w20213) -> (x-y*floor(x/y)=w20208:dbl, floor(x/y)=w20211:dbl)
                    n7790 = Quotient & Remainder(x=w20220, y=w20218) -> (x-y*floor(x/y)=w20215:dbl, floor(x/y)=w20219:dbl)
                    n7791 = Quotient & Remainder(x=w20211, y=w20213) -> (x-y*floor(x/y)=w20207:dbl, floor(x/y)=w20212:dbl)
                    n7792 = Quotient & Remainder(x=w20219, y=w20218) -> (x-y*floor(x/y)=w20214:dbl)  [unwired: 1 out]
                    n7793 = Quotient & Remainder(x=w20212, y=w20213) -> (x-y*floor(x/y)=w20206:dbl)  [unwired: 1 out]
                    n7794 = Build Array(w20214, w20215, w20216, w20217, w20206, w20207, w20208, w20209) -> (w20222:dbl[])
                  }
                  frame 4 {
                    w20229 = 256.0 ("y")
                    # "充电次数"
                    n7795 = Unbundle By Name(w20234) -> ("充电次数"=w20233:dbl, "应用车型"=w20231:dbl, "电池包组号"=w20230:dbl)
                    n7796 = Quotient & Remainder(x=w20233, y=w20229) -> (x-y*floor(x/y)=w20235:dbl, floor(x/y)=w20232:dbl)
                    n7797 = Quotient & Remainder(x=w20231, y=w20229) -> (x-y*floor(x/y)=w20227:dbl, floor(x/y)=w20228:dbl)
                    n7798 = Quotient & Remainder(x=w20230, y=w20229) -> (x-y*floor(x/y)=w20225:dbl, floor(x/y)=w20226:dbl)
                    n7799 = Build Array(w20232, w20235, w20228, w20227, w20226, w20225) -> (w20236:dbl[])
                  }
                  frame 5 {
                    # "SOC"
                    n7800 = Unbundle By Name(w20244) -> ("SOC"=w20243:dbl)
                    n7801 = call "输入分辨率计算-EV05.vi"("1字节?"=FALSE, "数值"=w20243, "分辨率"=0.1) -> ("低字节"=w20239:dbl, "高字节1"=w20240:dbl)  [unwired: 2 in, 5 out]
                    n7802 = Build Array(w20240, w20239) -> (w20245:dbl[])
                  }
                  frame 6 {
                    n7803 = Unbundle By Name(w20264) -> ("最大允许单体电压"=w20262:dbl, "最大允许总电压"=w20261:dbl, "最大允许温度"=w20260:dbl, "最小允许温度"=w20259:dbl, "最大允许充电电流"=w20258:dbl, "最小允许充电电流"=w20257:dbl, "电流步长"=w20253:dbl, "最小允许单体电压"=w20256:dbl)
                    n7804 = call "输入分辨率计算-EV05.vi"("1字节?"=FALSE, "数值 2"=w20256, "数值"=w20262, "分辨率"=0.001) -> ("低字节 2"=w20248:dbl, "高字节 2"=w20249:dbl, "低字节"=w20272:dbl, "高字节1"=w20273:dbl)  [unwired: 1 in, 3 out]
                    n7805 = call "输入分辨率计算-EV05.vi"("1字节?"=FALSE, "数值"=w20261, "分辨率"=0.1) -> ("低字节"=w20270:dbl, "高字节1"=w20271:dbl)  [unwired: 2 in, 5 out]
                    n7806 = call "输入分辨率计算-EV05.vi"("1字节?"=TRUE, "数值 2"=w20259, "数值"=w20260, "偏移量"=-40.0, "分辨率"=1.0) -> ("高字节 2"=w20265:dbl, "高字节1"=w20269:dbl)  [unwired: 5 out]
                    n7807 = call "输入分辨率计算-EV05.vi"("1字节?"=FALSE, "数值 2"=w20257, "数值"=w20258, "偏移量"=0.0, "分辨率"=0.1) -> ("低字节 2"=w20254:dbl, "高字节 2"=w20255:dbl, "低字节"=w20267:dbl, "高字节1"=w20268:dbl)  [unwired: 3 out]
                    n7808 = Quotient & Remainder(x=w20253, y=256.0) -> (x-y*floor(x/y)=w20250:dbl, floor(x/y)=w20251:dbl)
                    n7809 = Build Array(w20273, w20272, w20271, w20270, w20269, w20265, w20268, w20267, w20255, w20254, w20251, w20250, w20249, w20248) -> (w20266:dbl[])
                  }
                }
              }
            }
          }
        }
        frame "二维码" {
          w20296 = 30 ("长度")
          # "产品编号"
          n7810 = local read "从板二维码"() -> (w20285:string)
          n7811 = Search and Replace String(input string=w20285, search string="BNET" ("搜索字符串"), replace string="") -> (result string=w20291:string)  [unwired: 5 in, 3 out]
          n7812 = String To Byte Array(string=w20291) -> (unsigned byte array=w20294:u8[])
          n7813 = Array Subset(array=w20294, length=w20296) -> (w20298:u8[])  [unwired: 1 in]
          n7814 = Build Array(w20298) -> (w20290:u8[][])
          n7815 = Build Array(w20296) -> (w20288:i32[])
          n7816 = Build Array(u32 1 ("命令序号")) -> (w20287:u32[])
          n7817 = Build Array("写二维码") -> (w20289:string[])
        }
        frame "充电参数" {
          n7818 = case shown="真" w20303 {
            tunnel: [_ w20314] -> w20307
            tunnel: [_ w20313] -> w20306
            tunnel: w20305 -> [_ w20309]
            tunnel: [_ w20312] -> w20304
            tunnel: [_ u32 35 ("命令序号")] -> w20302
            frame False {
            }
            frame True {
              n7819 = Unbundle By Name(w20309) -> ("电池组信息(从板)"=w20310:refnum<vi>)
              n7820 = property class="Clust (严格)"(reference=w20310) -> ("Value"=w20308:T9)  [unwired: 1 in, 2 out]
              n7821 = for {
                N: 1 -> [_]
                tunnel: [w20320] -> w20314 mode=indexing
                tunnel: [w20319] -> w20313 mode=indexing
                tunnel: w20308 -> [w20318]
                tunnel: [w20317] -> w20312 mode=indexing
                i -> [w20316]
                n7822 = case shown="0, 默认" w20316 {
                  tunnel: [14 ("单个参数补充") 30 ("单个参数补充") 4 ("单个参数补充") 8 ("单个参数补充") 6 ("单个参数补充") 4 ("单个参数补充") 8 ("单个参数补充")] -> w20320
                  tunnel: [u32 7 ("命令序号") u32 1 ("命令序号") u32 2 ("命令序号") u32 3 ("命令序号") u32 4 ("命令序号") u32 5 ("命令序号") u32 6 ("命令序号")] -> w20319
                  tunnel: w20318 -> [w20337 w20373 w20386 w20393 w20422 w20432 w20439]
                  tunnel: [w20339 w20375 w20379 w20410 w20424 w20433 w20437] -> w20317
                  frame 0, Default {
                    n7823 = Unbundle By Name(w20337) -> ("最大允许单体电压"=w20335:dbl, "最大允许总电压"=w20334:dbl, "最大允许温度"=w20333:dbl, "最小允许温度"=w20332:dbl, "最大允许充电电流"=w20331:dbl, "最小允许充电电流"=w20330:dbl, "电流步长"=w20326:dbl, "最小允许单体电压"=w20329:dbl)
                    n7824 = call "输入分辨率计算-EV05.vi"("1字节?"=FALSE, "数值 2"=w20329, "数值"=w20335, "分辨率"=0.001) -> ("低字节 2"=w20321:dbl, "高字节 2"=w20322:dbl, "低字节"=w20345:dbl, "高字节1"=w20346:dbl)  [unwired: 1 in, 3 out]
                    n7825 = call "输入分辨率计算-EV05.vi"("1字节?"=FALSE, "数值"=w20334, "分辨率"=0.1) -> ("低字节"=w20343:dbl, "高字节1"=w20344:dbl)  [unwired: 2 in, 5 out]
                    n7826 = call "输入分辨率计算-EV05.vi"("1字节?"=TRUE, "数值 2"=w20332, "数值"=w20333, "偏移量"=-40.0, "分辨率"=1.0) -> ("高字节 2"=w20338:dbl, "高字节1"=w20342:dbl)  [unwired: 5 out]
                    n7827 = call "输入分辨率计算-EV05.vi"("1字节?"=FALSE, "数值 2"=w20330, "数值"=w20331, "偏移量"=0.0, "分辨率"=0.1) -> ("低字节 2"=w20327:dbl, "高字节 2"=w20328:dbl, "低字节"=w20340:dbl, "高字节1"=w20341:dbl)  [unwired: 3 out]
                    n7828 = Quotient & Remainder(x=w20326, y=256.0) -> (x-y*floor(x/y)=w20323:dbl, floor(x/y)=w20324:dbl)
                    n7829 = Build Array(w20346, w20345, w20344, w20343, w20342, w20338, w20341, w20340, w20328, w20327, w20324, w20323, w20322, w20321) -> (w20339:dbl[])
                  }
                  frame 1 {
                    w20363 = 0 ("索引")
                    # "电池组信息"
                    n7830 = Unbundle By Name(w20373) -> ("电池类型"=w20365:dbl, "电池厂家"=w20364:dbl, "电池厂家"=w20366:dbl, "电池类型"=w20367:dbl, "额定能量"=w20371:dbl, "额定容量"=w20368:dbl, "实际容量"=w20360:dbl)
                    n7831 = Build Array(w20365, w20364, w20363, w20363, w20363, w20363, w20363, w20366, w20367) -> (w20362:dbl[])
                    n7832 = call "输入分辨率计算-EV05.vi"("1字节?"=FALSE, "数值"=w20360, "分辨率"=0.1) -> ("高字节1"=w20358:dbl)  [unwired: 2 in, 6 out]
                    n7833 = Quotient & Remainder(x=w20371, y=256.0) -> (x-y*floor(x/y)=w20369:dbl, floor(x/y)=w20370:dbl)
                    n7834 = call "电池组信息组合.vi"("数组"=w20362) -> ("电池信息组合"=w20376:dbl[])
                    n7835 = Insert Into Array(array=w20376, index=0 ("索引"), new element #1=w20370, new element #2=w20369, new element #3=w20368, new element #4=w20358, new element #5=w20358) -> (w20375:dbl[])
                  }
                  frame 2 {
                    n7836 = Unbundle By Name(w20386) -> ("电池包序号"=w20383:dbl)
                    n7837 = Quotient & Remainder(x=w20383, y=256.0) -> (x-y*floor(x/y)=w20380:dbl, floor(x/y)=w20381:dbl)
                    n7838 = Build Array(w20381, w20380) -> (w20379:dbl[])
                  }
                  frame 3 {
                    w20401 = 256.0 ("y")
                    w20406 = 256.0 ("y")
                    # "充放电安时/安时数"
                    n7839 = Unbundle By Name(w20393) -> ("充电总安时"=w20390:dbl, "放电总这时"=w20389:dbl)
                    n7840 = call "输入分辨率计算-EV05.vi"("1字节?"=TRUE, "数值 2"=w20389, "数值"=w20390, "分辨率"=0.001) -> ("高字节 2"=w20387:dbl, "高字节1"=w20388:dbl)  [unwired: 1 in, 5 out]
                    n7841 = Quotient & Remainder(x=w20388, y=w20406) -> (x-y*floor(x/y)=w20405:dbl, floor(x/y)=w20409:dbl)
                    n7842 = Quotient & Remainder(x=w20387, y=w20401) -> (x-y*floor(x/y)=w20397:dbl, floor(x/y)=w20398:dbl)
                    n7843 = Quotient & Remainder(x=w20409, y=w20406) -> (x-y*floor(x/y)=w20404:dbl, floor(x/y)=w20408:dbl)
                    n7844 = Quotient & Remainder(x=w20398, y=w20401) -> (x-y*floor(x/y)=w20396:dbl, floor(x/y)=w20399:dbl)
                    n7845 = Quotient & Remainder(x=w20408, y=w20406) -> (x-y*floor(x/y)=w20403:dbl, floor(x/y)=w20407:dbl)
                    n7846 = Quotient & Remainder(x=w20399, y=w20401) -> (x-y*floor(x/y)=w20395:dbl, floor(x/y)=w20400:dbl)
                    n7847 = Quotient & Remainder(x=w20407, y=w20406) -> (x-y*floor(x/y)=w20402:dbl)  [unwired: 1 out]
                    n7848 = Quotient & Remainder(x=w20400, y=w20401) -> (x-y*floor(x/y)=w20394:dbl)  [unwired: 1 out]
                    n7849 = Build Array(w20402, w20403, w20404, w20405, w20394, w20395, w20396, w20397) -> (w20410:dbl[])
                  }
                  frame 4 {
                    w20417 = 256.0 ("y")
                    # "充电次数"
                    n7850 = Unbundle By Name(w20422) -> ("充电次数"=w20421:dbl, "应用车型"=w20419:dbl, "电池包组号"=w20418:dbl)
                    n7851 = Quotient & Remainder(x=w20421, y=w20417) -> (x-y*floor(x/y)=w20423:dbl, floor(x/y)=w20420:dbl)
                    n7852 = Quotient & Remainder(x=w20419, y=w20417) -> (x-y*floor(x/y)=w20415:dbl, floor(x/y)=w20416:dbl)
                    n7853 = Quotient & Remainder(x=w20418, y=w20417) -> (x-y*floor(x/y)=w20413:dbl, floor(x/y)=w20414:dbl)
                    n7854 = Build Array(w20420, w20423, w20416, w20415, w20414, w20413) -> (w20424:dbl[])
                  }
                  frame 5 {
                    # "SOC"
                    n7855 = Unbundle By Name(w20432) -> ("SOC"=w20431:dbl)
                    n7856 = call "输入分辨率计算-EV05.vi"("1字节?"=FALSE, "数值"=w20431, "分辨率"=0.1) -> ("低字节"=w20427:dbl, "高字节1"=w20428:dbl)  [unwired: 2 in, 5 out]
                    n7857 = Build Array(w20428, w20427) -> (w20433:dbl[])
                  }
                  frame 6 {
                    # "车牌号"
                    n7858 = Unbundle By Name(w20439) -> ("车牌号"=w20438:string)
                    n7859 = String To Byte Array(string=w20438) -> (unsigned byte array=w20442:u8[])
                    n7860 = Array Subset(array=w20442, length=8 ("长度")) -> (w20437:u8[])  [unwired: 1 in]
                  }
                }
              }
            }
          }
        }
      }
    }
  }
  "输出数组" <- w9
  "命令序号" <- w8
  "数组长度" <- w7
  "命令" <- w6
  "循环次数" <- w2
  "名称" <- w1
